vi "RT_Main.vi"() -> ()   [LabVIEW 2016]
uses:
  support/InputSelector.ctl
panel:
  in  "Input Method":T1
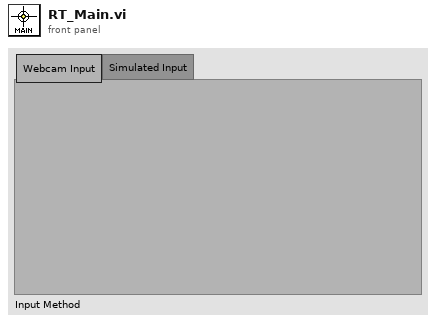
[diagram p1: front panel]
types:
  T1 = typedef "InputSelector.ctl" = enum32{"Webcam Input", "Simulated Input"}
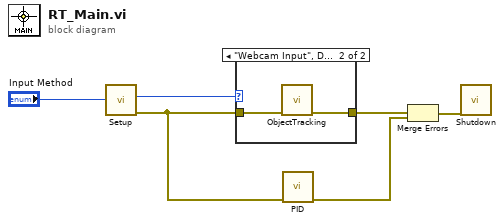
[diagram p0: block diagram]
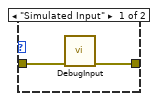
[diagram p2: hidden frame]
diagram:
  n1 = call "Setup.vi"("Input Method In"="Input Method") -> ("error out"=w4:errorcluster, "Input Method In 2"=w6:T1)  [unwired: 9 in]
  n2 = case shown="\"Webcam Input\", Default" w6 {
    tunnel: w4 -> [w8 w10]
    tunnel: [w7 w9] -> w2
    frame "Simulated Input" {
      n3 = call "DebugInput.vi"("error in (no error)"=w8) -> ("error out"=w7:errorcluster)  [unwired: 7 in, 2 out]
    }
    frame "Webcam Input", Default {
      n4 = call "ObjectTracking.vi"("error in"=w10) -> ("error out"=w9:errorcluster)  [unwired: 8 in, 1 out]
    }
  }
  n5 = call "PID.vi"("error in (no error)"=w4) -> ("error out"=w1:errorcluster)  [unwired: 8 in, 2 out]
  n6 = Merge Errors(w2, w1) -> (w3:errorcluster)
  n7 = call "Shutdown.vi"("error in (no error)"=w3) -> ()  [unwired: 11 in]
